vi "Format Error.vi"(8 "error in (no error)":errorcluster, 10 "Message":string, 11 "Error Type":T1) -> (0 "error out":errorcluster)   [LabVIEW 2020, in "LINX API.lvclass"]
uses:
  LINX API.lvclass
  LINX API.lvclass/LINX API.ctl
  Private/Type Defs/Error Type.ctl
  LMH-LINX.lvlib
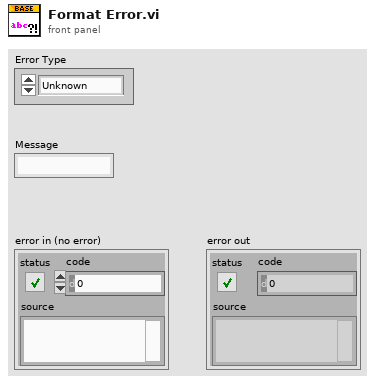
[diagram p1: front panel]
types:
  T1 = typedef "LMH-LINX.lvlib/Error Type.ctl" = enum16{"Unknown", "Timeout", "Corrupt Return Packet", "Unable To Connect", "Command Not Supported", "Channel DNE", "Invalid COM Config", "Firmware Version Mismatch", "myRIO Support", "CMD Specific Error", "Local IO Not Supported"}
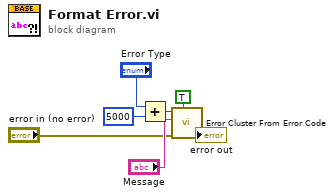
[diagram p0: block diagram]
diagram:
  n1 = Add(x="Error Type", y=5000) -> (x+y=w4:i32)
  n2 = call <vilib>:"Error Cluster From Error Code.vi"("show call chain? (False)"=TRUE, "error in (no error)"="error in (no error)", "error message (\"\")"="Message", "error code (0)"=w4) -> ("error out"=→"error out":errorcluster)  [unwired: 5 in]
